vi "Get Names.vi"(8 "error in (no error)":errorcluster, 11 "Session Handle in":T1) -> (0 "error out":errorcluster, 2 "Metric Names":string[](array[string]), 3 "Session Handle out":T1)   [LabVIEW 2020, in "Registry.lvlib" / "Registry Session.lvclass"]
uses:
  Registry Session.lvclass
  Typedefs/Session Handle.ctl
  Registry Session.lvclass/Registry Session.ctl
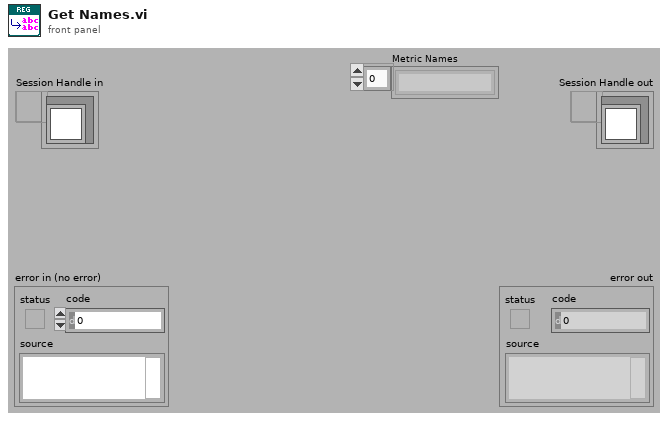
[diagram p1: front panel]
types:
  T1 = typedef "Registry.lvlib/Registry Session.lvclass/Session Handle.ctl" = refnum<data-value>
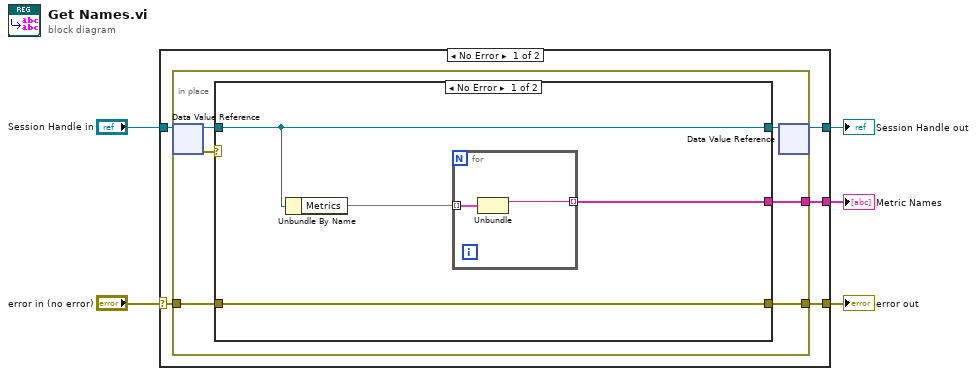
[diagram p0: block diagram]
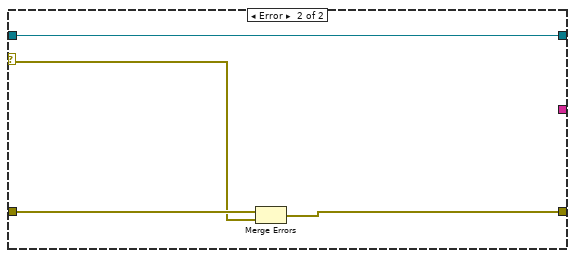
[diagram p2: hidden frame]
diagram:
  n1 = case shown="No Error" "error in (no error)" {
    selector: "error in (no error)" -> [w8 w27]
    tunnel: "Session Handle in" -> [w10 w28]
    tunnel: [w9 w28] -> w4
    tunnel: [w7 w27] -> w3
    tunnel: [w6 _] -> w1
    frame No Error {
      n2 = in-place {
        in-place-border: w8 -> [w12]
        in-place-border: [w15] -> w7
        in-place-border: [w11] -> w6
        n3 = in-place-dvr #1(w10) -> (w16:refnum<class "Registry Session.lvclass">, w13:errorcluster)
        n4 = case shown="No Error" w13 {
          selector: w13 -> [_ w25]
          tunnel: w16 -> [w19 w23]
          tunnel: [w20 w24] -> w15
          tunnel: [w19 w23] -> w14
          tunnel: w12 -> [w20 w26]
          tunnel: [w17 _] -> w11
          frame No Error {
            n5 = Unbundle By Name(w19) -> ("Metrics"=w18:map{string, refnum<data-value>})
            n6 = for {
              tunnel: w18 -> [w22] mode=indexing
              tunnel: [w21] -> w17 mode=indexing
              n7 = Unbundle(w22) -> (w21:string)  [unwired: 1 out]
            }
          }
          frame Error {
            n8 = Merge Errors(w26, w25) -> (w24:errorcluster)
          }
        }
        n9 = in-place-dvr #1(w14) -> (w9:T1)  [unwired: 1 out]
      }
    }
    frame Error {
    }
  }
  "Session Handle out" <- w4
  "error out" <- w3
  "Metric Names" <- w1
